vi "Write Scale.vi"(5 "Scale":refnum<class "Scale.lvclass">, 9 "Slide in":refnum<class "Slide.lvclass">) -> (3 "Slide out":refnum<class "Slide.lvclass">)   [LabVIEW 2014, in "Raspberry Pi Compatible Compiler for LabVIEW.lvlib" / "Slide.lvclass"]
uses:
  Slide.lvclass
  Scale/Scale.lvclass
  Slide.lvclass/Slide.ctl
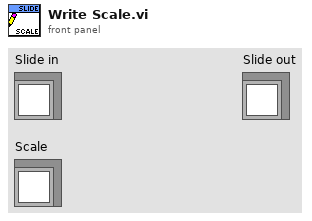
[diagram p1: front panel]
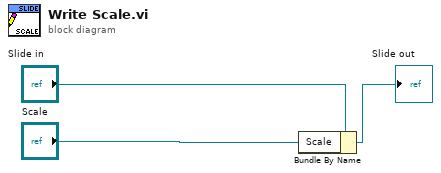
[diagram p0: block diagram]
diagram:
  n1 = Bundle By Name(cluster="Slide in", "Scale"="Scale") -> (→"Slide out":refnum<class "Slide.lvclass">)
